vi "sequencerHandshakes.vi"   [LabVIEW 2014]
uses:
  <vilib>/Platform/TimedLoop/XDataNode/timing_clust.ctl
  <vilib>/Platform/TimedLoop/XDataNode/nitl_modes.ctl
  <vilib>/Platform/TimedLoop/XDataNode/wakeup.ctl
  <vilib>/rvi/Emulation/niFpgaSctlEmulationGetInTimedLoop.vi
  <vilib>/rvi/Emulation/niFpgaEmulationReportErrorSimple.vi
  <vilib>/rvi/Emulation/niFpgaGetClockAttributes.vi
  <vilib>/rvi/Emulation/niFpgaCriticalErrorInLSC.vi
  <vilib>/rvi/Emulation/niFpgaEmulationIsFPGAContextNoSignature.vi
  <vilib>/rvi/DataTransferAndStorage/Container/Common/niFpgaContainerGetUniqueNameForEmu.vi
  <vilib>/rvi/eio/common/nirviEmuReportErrorAndStop.vi
  <vilib>/rvi/Emulation/niFpgaProcessEmulError.vi
  sequencerGlobVars.vi
  <vilib>/Platform/TimedLoop/XDataNode/XDataNode.xnode
  <vilib>/rvi/DataTransferAndStorage/Container/XNode/niFpgaContainer.xnode
  <vilib>/rvi/DataTransferAndStorage/Handshake/Emulation/niFpgaHandshakeEmulation.vi
  <vilib>/Platform/TimedLoop/XDataNode/XDNodeRunTimeDep.lvlib
types:
  T1 = typedef "XDNodeRunTimeDep.lvlib/timing_clust.ctl" = cluster{"Expected End [f-1]":u64, "Actual End [f-1]":u64, "Finished Late? [f-1]":bool, "Expected End [i-1]":u64, "Actual End [i-1]":u64, "Finished Late? [i-1]":bool, "Expected Start [i]":u64, "Actual Start [i]":u64, "Expected Start [f]":u64, "Actual Start [f]":u64, "Source Name":string, "Structure Name":string, "Period":i64, "Deadline":i64, "Offset":i64, "Start":i64, "Priority":i32, "Timeout":i32, "Mode":T2, "Wakeup Reason":T3, "Error":errorcluster, "Source Type":string, "Secondary Source Type":string, "Global End Time":u64, "Global Start Time":u64, "Frame Duration":u64, "Iteration Duration":u64, "Assigned CPU":i32, "I/O Scan Engine Mode":u32}
  T2 = typedef "XDNodeRunTimeDep.lvlib/nitl_modes.ctl" = enum32{"No Change", "Process missed periods, maintain original phase", "Discard missed periods, maintain original phase", "Process missed periods, ignore original phase", "Discard missed periods, ignore original phase"}
  T3 = typedef "XDNodeRunTimeDep.lvlib/wakeup.ctl" = enum32{"Normal", "Aborted", "Asynchronous wakeup", "Timing source error", "Timed loop error", "Timeout"}
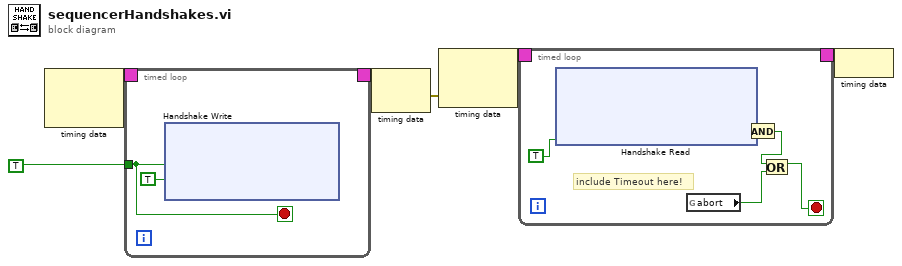
[diagram p0: block diagram]
diagram:
  n1 = node-c288() -> (w6:T1)  [unwired: 2 in]
  n2 = timed-loop {
    timing: w6 -> [_]
    timing-out: [_] -> w5
    tunnel: TRUE -> [w7]
    stop <- w7 stop-if-true
    n3 = xnode "Handshake Write"("Data"=w7, "Input Valid"=TRUE) -> ()  [unwired: 1 in, 2 out]
  }
  n4 = node-c288(w5) -> (w2:errorcluster)
  n5 = node-c288(w2) -> (w4:T1)  [unwired: 1 in]
  n6 = timed-loop {
    timing: w4 -> [_]
    timing-out: [_] -> w3
    stop <- w12 stop-if-true
    # "include Timeout here!"
    n7 = xnode "Handshake Read"("Ready for Output"=TRUE) -> ("Data"=w15:bool, "Output Valid"=w14:bool)  [unwired: 1 in, 1 out]
    n8 = global read "sequencerGlobVars.vi" "abort"() -> (w11:bool)
    n9 = And(x=w15, y=w14) -> (x .and. y?=w16:bool)
    n10 = Or(x=w16, y=w11) -> (x .or. y?=w12:bool)
  }
  n11 = node-c288(w3) -> ()
